vi "Platine Prog.vi"() -> ()   [LabVIEW 2024]
uses:
  Newport.SMC100.CommandInterface
panel:
  out "error out":errorcluster
  in  "Reset":bool
  out "StageIdentifier":string
  out "ConfigurationMode":i32
  out "ControllerVersion":string
  out "Instrument Key OUT":string
  out "controllerState":string
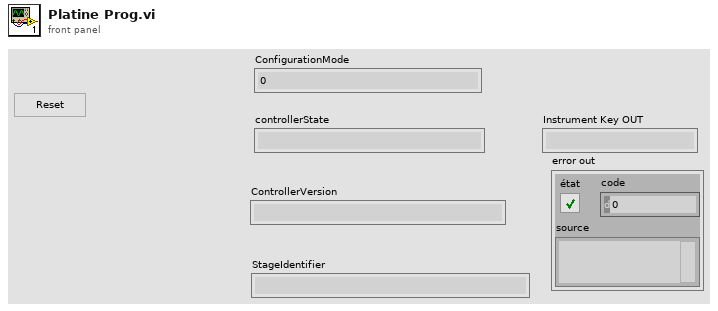
[diagram p1: front panel]
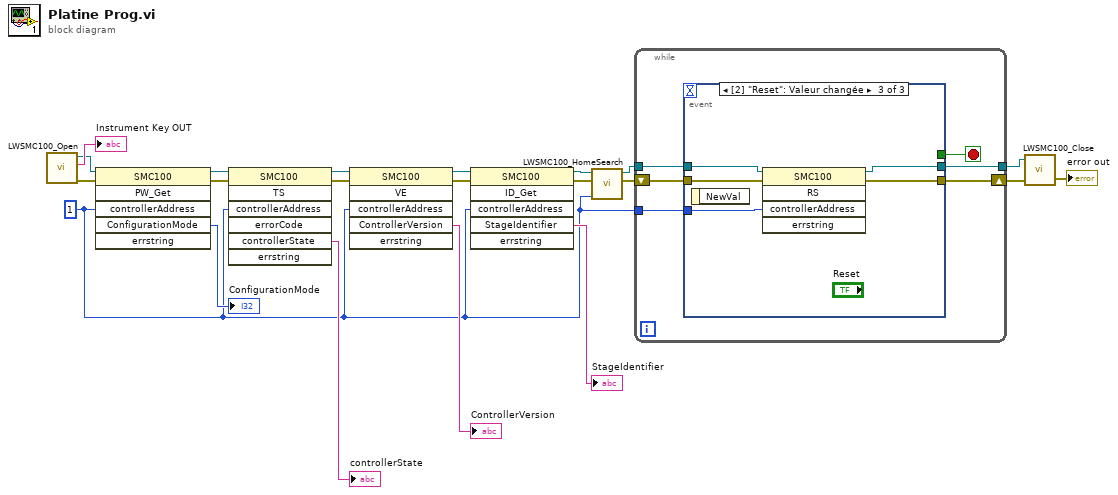
[diagram p0: block diagram]
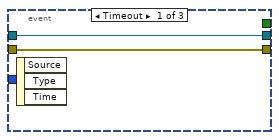
[diagram p2: hidden frame]
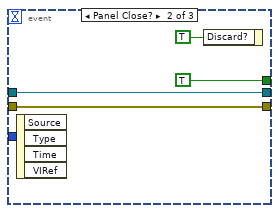
[diagram p3: hidden frame]
diagram:
  w1 = 1 ("controllerAddress IN")
  n1 = call "LWSMC100_Open.vi"() -> ("error out"=w15:errorcluster, "Instrument Key OUT"=→"Instrument Key OUT":string, "CommandInterfaceSMC100.SMC100"=w13:refnum<k24>)  [unwired: 4 in, 1 out]
  n2 = invoke on="Nœud de méthode" class="SMC100" method="PW_Get"(reference=w13, error in=w15, "controllerAddress"=w1) -> (reference out=w12:refnum<k24>, error out=w14:errorcluster, "ConfigurationMode"=→"ConfigurationMode":i32)  [unwired: 3 in, 3 out]
  n3 = invoke on="Nœud de méthode" class="SMC100" method="TS"(reference=w12, error in=w14, "controllerAddress"=w1) -> (reference out=w19:refnum<k24>, error out=w18:errorcluster, "controllerState"=→"controllerState":string)  [unwired: 4 in, 4 out]
  n4 = invoke on="Nœud de méthode" class="SMC100" method="VE"(reference=w19, error in=w18, "controllerAddress"=w1) -> (reference out=w9:refnum<k24>, error out=w11:errorcluster, "ControllerVersion"=→"ControllerVersion":string)  [unwired: 3 in, 3 out]
  n5 = invoke on="Nœud de méthode" class="SMC100" method="ID_Get"(reference=w9, error in=w11, "controllerAddress"=w1) -> (reference out=w7:refnum<k24>, error out=w8:errorcluster, "StageIdentifier"=→"StageIdentifier":string)  [unwired: 3 in, 3 out]
  n6 = call "LWSMC100_HomeSearch.vi"("controllerAddress IN"=w1, "Error IN"=w8, "CommandInterfaceSMC100.SMC100"=w7) -> ("error out"=w6:errorcluster, "CommandInterfaceSMC100.SMC100"=w2:refnum<k24>)  [unwired: 4 in, 3 out]
  n7 = while {
    tunnel: [w24] -> w3
    tunnel: w2 -> [w23]
    shift-right: [w26] -> w5
    shift-left: w6 -> [w25]
    tunnel: w1 -> [w22]
    stop <- w27 stop-if-true
    n8 = event shown="[2] \"Reset\": Valeur changée" {
      selector: _ -> [_ _ _]
      dyn-events: _ -> [_ _ _]
      timeout: _ -> [_ _ _]
      tunnel: [_ TRUE ("Rejeter ?") _] -> w27
      tunnel: [w28 w31 w37] -> w26
      tunnel: w25 -> [w28 w31 w38]
      tunnel: [w29 w30 w35] -> w24
      tunnel: w23 -> [w29 w30 w36]
      tunnel: w22 -> [_ _ w34]
      event Timeout {
        n9 = event-data() -> ()  [unwired: 1 in, 3 out]
      }
      event Panel Close? {
        n10 = event-data() -> ()  [unwired: 1 in, 4 out]
        n11 = event-data("Discard?"=TRUE ("Rejeter ?")) -> ()  [unwired: 1 in, 1 out]
      }
      event "Reset": Value Change {
        n12 = event-data() -> ()  [unwired: 1 in, 1 out]
        n13 = invoke on="Nœud de méthode" class="SMC100" method="RS"(reference=w36, error in=w38, "controllerAddress"=w34) -> (reference out=w35:refnum<k24>, error out=w37:errorcluster)  [unwired: 2 in, 3 out]
      }
    }
  }
  n14 = call "LWSMC100_Close.vi"("error in (no error)"=w5, "CommandInterfaceSMC100.SMC100"=w3) -> ("Error out"=→"error out":errorcluster)  [unwired: 1 in, 1 out]
